vi "PID Least Square.vi"(0 "Double integral delta Y":dbl[](array[numeric]), 2 "TF order":enum16{"1st Order", "2nd Order"}(ring), 3 "with delay?":bool, 5 "Integral delta Y":dbl[](array[numeric]), 7 "Delta Y":dbl[](array[numeric]), 9 "Time array":dbl[](array[numeric]), 13 "Inverse response?":bool) -> (4 "Delay":dbl, 6 "b1":dbl, 8 "b2":dbl, 10 "a0":dbl)   [LabVIEW 2020, in "NI_PID_autopid.lvlib"]
uses:
  <vilib>/addons/control/pid/NI_PID_autopid.lvlib
  <vilib>/Analysis/baseanly.llb/Real Dot Product.vi
  <vilib>/Analysis/baseanly.llb/Real A x B.vi
  <vilib>/Analysis/baseanly.llb/A x Vector.vi
  <vilib>/Analysis/baseanly.llb/Real Inverse Matrix.vi
  <vilib>/Analysis/NI_AALBase.lvlib
panel:
  out "error":bool
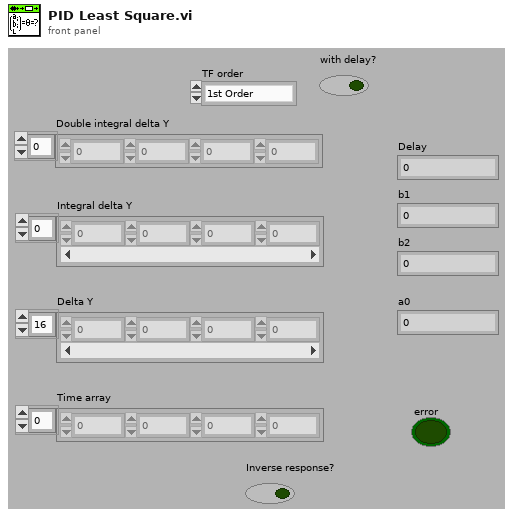
[diagram p1: front panel]
types:
  T1 = typedef "NI_Matrix.lvlib/RealMatrix.ctl" = dbl[][]
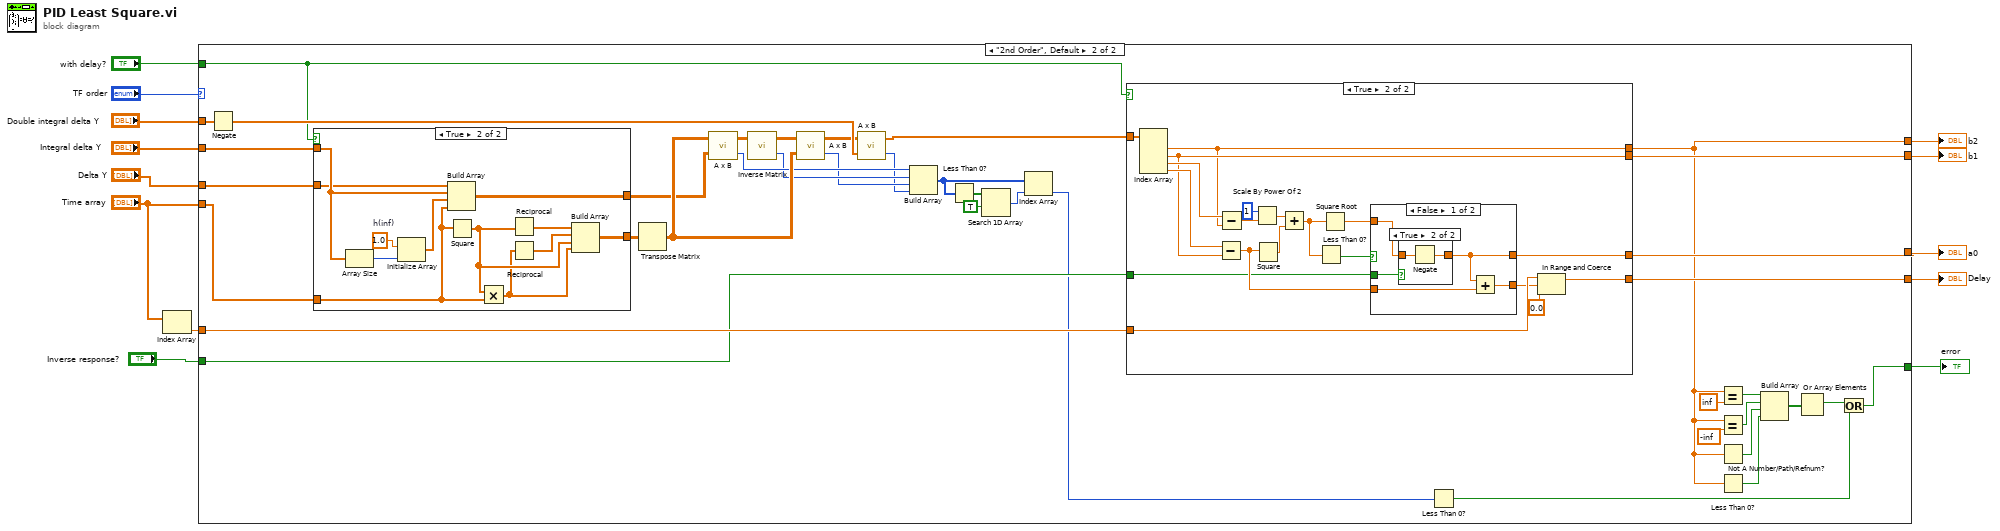
[diagram p0: block diagram]
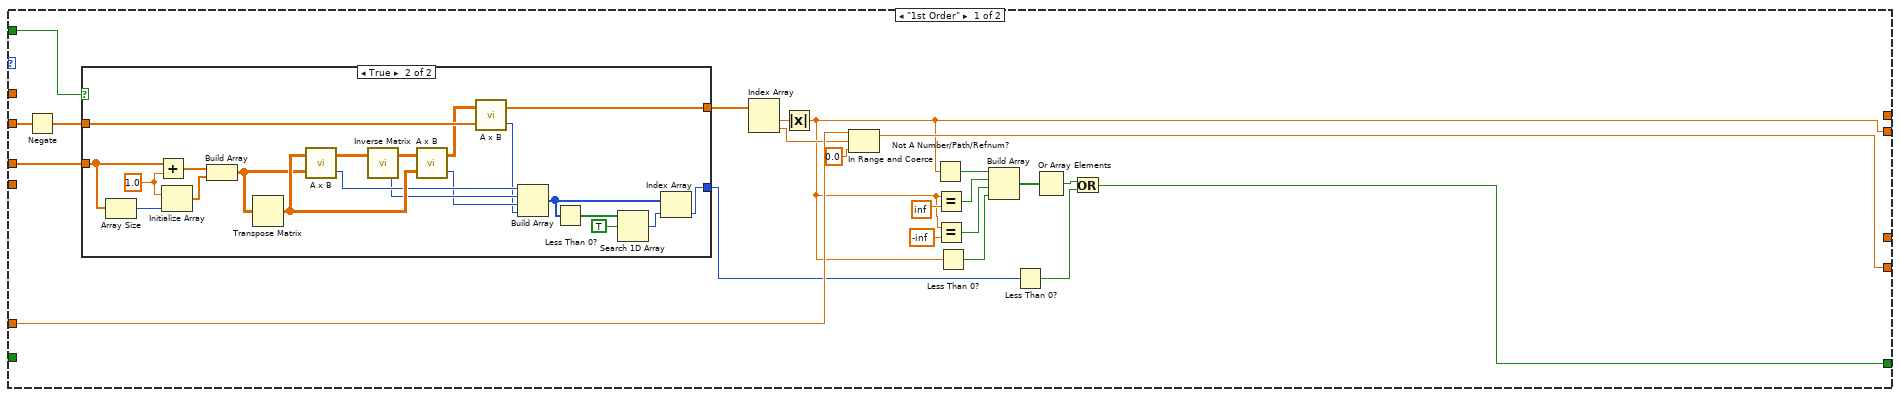
[diagram p2: hidden frame]
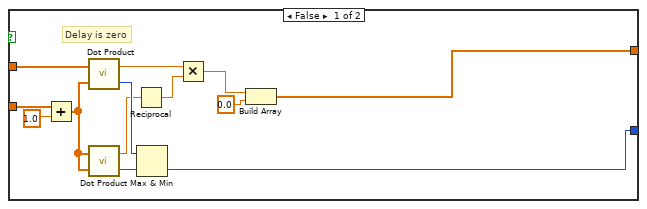
[diagram p3: hidden frame]
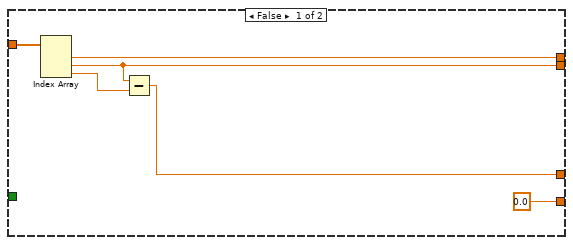
[diagram p4: hidden frame]
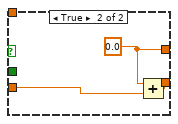
[diagram p6: hidden frame]
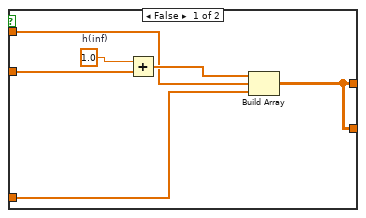
[diagram p7: hidden frame]
diagram:
  n1 = Index Array(array="Time array") -> (element=w1:dbl)  [unwired: 1 in]
  n2 = case shown="\"2nd Order\", Default" "TF order" {
    tunnel: "Delta Y" -> [w29 w101]
    tunnel: "Integral delta Y" -> [w35 w100]
    tunnel: w1 -> [w34 w102]
    tunnel: "Double integral delta Y" -> [_ w103]
    tunnel: "Time array" -> [_ w99]
    tunnel: "Inverse response?" -> [_ w98]
    tunnel: [w17 w74] -> w7
    tunnel: "with delay?" -> [w28 w94]
    tunnel: [w14 w72] -> w5
    tunnel: [_ w73] -> w4
    tunnel: [_ w71] -> w3
    tunnel: [w15 w70] -> w2
    frame "1st Order" {
      n3 = Negate(x=w35) -> (-x=w30:dbl[])
      n4 = case shown="True" w28 {
        tunnel: [w44 w68] -> w33
        tunnel: [w43 w66] -> w16
        tunnel: w30 -> [w48 w65]
        tunnel: w29 -> [w47 w64]
        frame False {
          # "Delay is zero"
          n5 = Add(x=w47, y=1.0) -> (x+y=w38:dbl[])
          n6 = call-poly <vilib>:"Dot Product.vi"("Y Vector"=w38, "X Vector"=w48) -> ("error"=w41:i32, "X * Y"=w39:dbl)
          n7 = call-poly <vilib>:"Dot Product.vi"("Y Vector"=w38, "X Vector"=w38) -> ("error"=w42:i32, "X * Y"=w37:dbl)
          n8 = Reciprocal(x=w37) -> (1/x=w40:dbl)
          n9 = Max & Min(x=w41, y=w42) -> (min(x,y)=w43:i32)  [unwired: 1 out]
          n10 = Multiply(x=w39, y=w40) -> (x*y=w46:dbl)
          n11 = Build Array(w46, 0.0 ("element")) -> (w44:dbl[])
        }
        frame True {
          w62 = 1.0 ("h(inf)")
          n12 = Array Size(array=w64) -> (size(s)=w61:i32)
          n13 = Add(x=w64, y=w62) -> (x+y=w63:dbl[])
          n14 = Initialize Array(w62, w61) -> (w60:dbl[])
          n15 = Build Array(w63, w60) -> (w67:T1)
          n16 = Transpose Matrix(1:w67) -> (0:w69:T1)
          n17 = call-poly <vilib>:"A x B.vi"("B"=w67, "A"=w69) -> ("error"=w56:i32, "A x B"=w59:T1)
          n18 = call-poly <vilib>:"Inverse Matrix.vi"("Input Matrix"=w59) -> ("error"=w55:i32, "Inverse Matrix"=w58:T1)  [unwired: 1 in]
          n19 = call-poly <vilib>:"A x B.vi"("B"=w69, "A"=w58) -> ("error"=w54:i32, "A x B"=w57:T1)
          n20 = call-poly <vilib>:"A x B.vi"("Vector"=w65, "A"=w57) -> ("error"=w53:i32, "A x Vector"=w68:dbl[])
          n21 = Build Array(w56, w55, w54, w53) -> (w50:i32[])
          n22 = Less Than 0?(x=w50) -> (x < 0?=w52:bool[])
          n23 = Search 1D Array(1D array=w52, element=TRUE) -> (index of element=w49:i32)  [unwired: 1 in]
          n24 = Index Array(array=w50, index=w49) -> (element=w66:i32)
        }
      }
      n25 = Index Array(array=w33) -> (element #1=w18:dbl, element #2=w20:dbl)  [unwired: 2 in]
      n26 = Absolute Value(x=w18) -> (abs(x)=w14:dbl)
      n27 = In Range and Coerce(upper limit=w34, x=w20, lower limit=0.0) -> (coerced(x)=w17:dbl)  [unwired: 1 out]
      n28 = Not A Number/Path/Refnum?(number/path/refnum=w14) -> (NaN/Path/Refnum?=w23:bool)
      n29 = Equal?(x=w14, y=inf ("x")) -> (x = y?=w24:bool)
      n30 = Equal?(x=w14, y=-inf) -> (x = y?=w25:bool)
      n31 = Less Than 0?(x=w14) -> (x < 0?=w27:bool)
      n32 = Build Array(w23, w24, w25, w27) -> (w26:bool[])
      n33 = Less Than 0?(x=w16) -> (x < 0?=w31:bool)
      n34 = Or Array Elements(Boolean array=w26) -> (logical OR=w32:bool)
      n35 = Or(x=w32, y=w31) -> (x .or. y?=w15:bool)
    }
    frame "2nd Order", Default {
      n36 = Negate(x=w103) -> (-x=w105:dbl[])
      n37 = case shown="True" w94 {
        tunnel: w100 -> [w146 w160]
        tunnel: w101 -> [w148 w159]
        tunnel: w99 -> [w145 w158]
        tunnel: [w144 w153] -> w104
        tunnel: [w144 w152] -> w93
        frame False {
          w147 = 1.0  # h(inf)
          n38 = Add(x=w147, y=w148) -> (x+y=w149:dbl[])
          n39 = Build Array(w149, w146, w145) -> (w144:T1)
        }
        frame True {
          w151 = 1.0  # h(inf)
          n40 = Array Size(array=w160) -> (size(s)=w161:i32)
          n41 = Initialize Array(w151, w161) -> (w150:dbl[])
          n42 = Build Array(w159, w160, w150, w158) -> (w153:T1)
          n43 = Square(x=w158) -> (x^2=w155:dbl[])
          n44 = Multiply(x=w155, y=w158) -> (x*y=w154:dbl[])
          n45 = Reciprocal(x=w155) -> (1/x=w157:dbl[])
          n46 = Reciprocal(x=w154) -> (1/x=w156:dbl[])
          n47 = Build Array(w157, w156, w155, w154) -> (w152:T1)
        }
      }
      n48 = Transpose Matrix(1:w93) -> (0:w107:T1)
      n49 = call-poly <vilib>:"A x B.vi"("B"=w104, "A"=w107) -> ("error"=w89:i32, "A x B"=w92:T1)
      n50 = call-poly <vilib>:"Inverse Matrix.vi"("Input Matrix"=w92) -> ("error"=w88:i32, "Inverse Matrix"=w91:T1)  [unwired: 1 in]
      n51 = call-poly <vilib>:"A x B.vi"("B"=w107, "A"=w91) -> ("error"=w87:i32, "A x B"=w90:T1)
      n52 = call-poly <vilib>:"A x B.vi"("Vector"=w105, "A"=w90) -> ("error"=w86:i32, "A x Vector"=w106:dbl[])
      n53 = Build Array(w89, w88, w87, w86) -> (w83:i32[])
      n54 = Less Than 0?(x=w83) -> (x < 0?=w85:bool[])
      n55 = Search 1D Array(1D array=w85, element=TRUE) -> (index of element=w82:i32)  [unwired: 1 in]
      n56 = Index Array(array=w83, index=w82) -> (element=w95:i32)
      n57 = case shown="True" w94 {
        tunnel: w106 -> [w113 w132]
        tunnel: w98 -> [_ w121]
        tunnel: w102 -> [_ w120]
        tunnel: [0.0 ("T1") w117] -> w74
        tunnel: [w110 w116] -> w73
        tunnel: [w108 w114] -> w71
        tunnel: [w109 w115] -> w72
        frame False {
          n58 = Index Array(array=w113) -> (element #1=w108:dbl, element #2=w109:dbl, element #3=w112:dbl)  [unwired: 3 in]
          n59 = Subtract(x=w109, y=w112) -> (x-y=w110:dbl)
        }
        frame True {
          n60 = Index Array(array=w132) -> (element #1=w114:dbl, element #2=w115:dbl, element #3=w131:dbl, element #4=w128:dbl)  [unwired: 4 in]
          n61 = Subtract(x=w128, y=w115) -> (x-y=w122:dbl)
          n62 = Subtract(x=w131, y=w114) -> (x-y=w130:dbl)
          n63 = Scale By Power Of 2(n=1, x=w130) -> (x*2^n=w127:dbl)
          n64 = Square(x=w122) -> (x^2=w126:dbl)
          n65 = Add(x=w127, y=w126) -> (x+y=w125:dbl)
          n66 = Less Than 0?(x=w125) -> (x < 0?=w123:bool)
          n67 = Square Root(x=w125) -> (sqrt(x)=w124:dbl)
          n68 = case shown="False" w123 {
            tunnel: w124 -> [w136 _]
            tunnel: [w134 w143] -> w116
            tunnel: w122 -> [w135 w142]
            tunnel: w121 -> [w137 _]
            tunnel: [w133 w141] -> w118
            frame False {
              n69 = case shown="True" w137 {
                tunnel: w136 -> [w138 w140]
                tunnel: [w138 w139] -> w134
                frame False {
                }
                frame True {
                  n70 = Negate(x=w140) -> (-x=w139:dbl)
                }
              }
              n71 = Add(x=w134, y=w135) -> (x+y=w133:dbl)
            }
            frame True {
              w143 = 0.0
              n72 = Add(x=w143, y=w142) -> (x+y=w141:dbl)
            }
          }
          n73 = In Range and Coerce(upper limit=w120, x=w118, lower limit=0.0) -> (coerced(x)=w117:dbl)  [unwired: 1 out]
        }
      }
      n74 = Less Than 0?(x=w95) -> (x < 0?=w96:bool)
      n75 = Equal?(x=w71, y=inf ("element")) -> (x = y?=w77:bool)
      n76 = Equal?(x=w71, y=-inf ("element")) -> (x = y?=w78:bool)
      n77 = Not A Number/Path/Refnum?(number/path/refnum=w71) -> (NaN/Path/Refnum?=w79:bool)
      n78 = Less Than 0?(x=w71) -> (x < 0?=w80:bool)
      n79 = Build Array(w77, w78, w79, w80) -> (w81:bool[])
      n80 = Or Array Elements(Boolean array=w81) -> (logical OR=w97:bool)
      n81 = Or(x=w97, y=w96) -> (x .or. y?=w70:bool)
    }
  }
  "Delay" <- w7
  "b1" <- w5
  "a0" <- w4
  "b2" <- w3
  "error" <- w2
